vi "Write AGAINx.vi"(8 "error in (no error)":errorcluster, 10 "AGAINx":i32, 11 "AMS TS3472 in":refnum<class "AMS TCS3472.lvclass">) -> (0 "error out":errorcluster, 3 "AMS TS3472 out":refnum<class "AMS TCS3472.lvclass">)   [LabVIEW 2014, in "AMS TS3472 Light Sensor.lvlib" / "AMS TCS3472.lvclass"]
uses:
  AMS TCS3472.lvclass
  AMS TCS3472.lvclass/AMS TCS3472.ctl
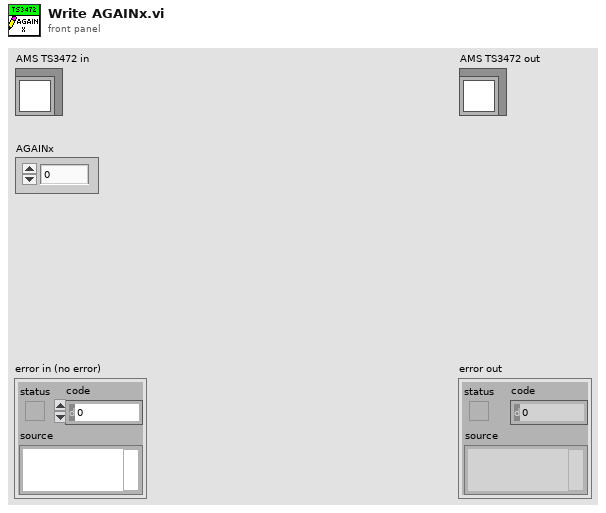
[diagram p1: front panel]
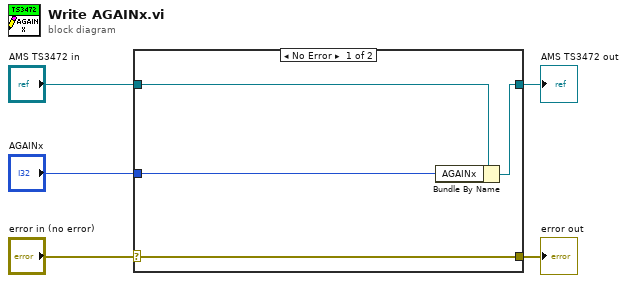
[diagram p0: block diagram]
diagram:
  n1 = case shown="No Error" "error in (no error)" {
    selector: "error in (no error)" -> [w9 w10]
    tunnel: [w9 w10] -> w4
    tunnel: [w7 w11] -> w2
    tunnel: "AMS TS3472 in" -> [w8 w11]
    tunnel: "AGAINx" -> [w6 _]
    frame No Error {
      n2 = Bundle By Name(cluster=w8, "AGAINx"=w6) -> (w7:refnum<class "AMS TCS3472.lvclass">)
    }
    frame Error {
    }
  }
  "error out" <- w4
  "AMS TS3472 out" <- w2
